vi "DataPathDialog.vi"(11 "Path":path=path "click on the folder icon to choose a folder") -> (1 "canceled?":bool, 3 "Path out":path)   [LabVIEW 2022 SP3]
panel:
  in  "Cancel Button":bool
  in  "OK Button":bool
  # "Welcome to Oberlin Acoustics \nacquiring data from a violin"
  # "1. Select your Data Folder\n       this is the folder for all your data"
  # "2. Check out directions\n       understand where to get help"
  # "https://sites.google.com/view/oberlinacoustics"
  # "3. Getting Started\n       First time users should hit the Getting     \n       Started button on the next screen (after \n       clicking on OK)"
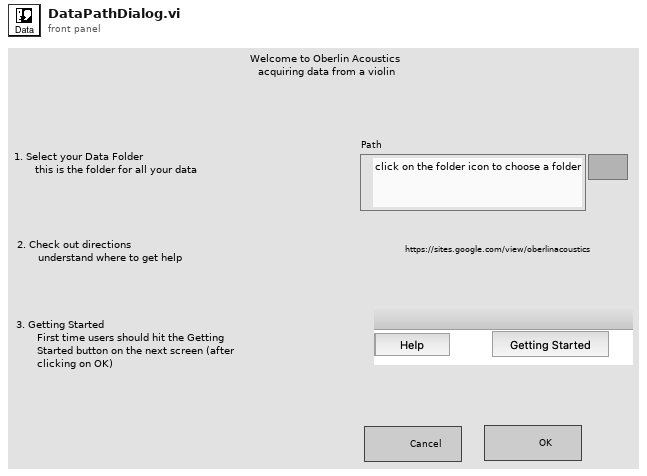
[diagram p1: front panel]
types:
  T1 = enum8{"Enabled", "Disabled", "Disabled and Grayed Out"}
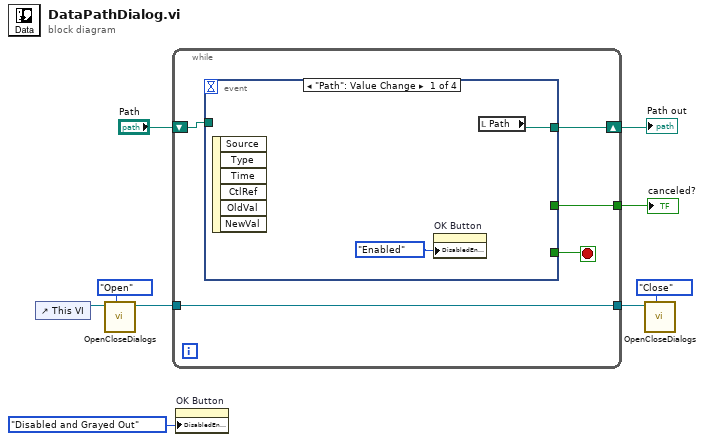
[diagram p0: block diagram]
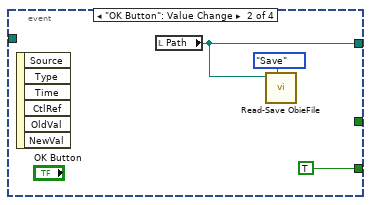
[diagram p2: hidden frame]
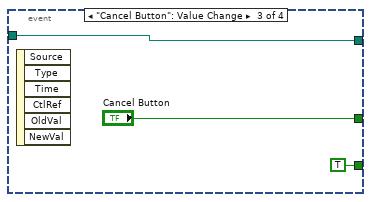
[diagram p3: hidden frame]
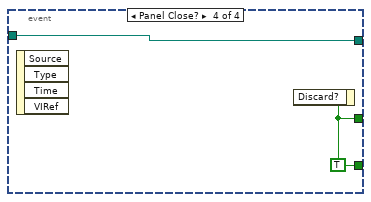
[diagram p4: hidden frame]
diagram:
  n1 = control-ref of="This VI"() -> (w4:refnum<vi>)
  n2 = call "OpenCloseDialogs.vi"("Task"=enum16{"Open", "Close"}."Open", "VI in"=w4) -> ("VI out"=w1:refnum<vi>)  [unwired: 8 in, 1 out]
  n3 = while {
    shift-right: [w12] -> w9
    shift-left: "Path" -> [w14]
    tunnel: [w11] -> w7
    tunnel: [w10] -> w2
    tunnel: w1 -> [w10]
    stop <- w13 stop-if-true
    n4 = event shown="[0] \"Path\": Value Change" {
      selector: _ -> [_ _ _ _]
      dyn-events: _ -> [_ _ _ _]
      timeout: _ -> [_ _ _ _]
      tunnel: [w16 w19 w22 w24] -> w12
      tunnel: w14 -> [_ _ w22 w24]
      tunnel: [_ TRUE TRUE w23] -> w13
      tunnel: [_ _ "Cancel Button" w23] -> w11
      event "Path": Value Change {
        n5 = event-data() -> ()  [unwired: 1 in, 6 out]
        n6 = property on="OK Button" class="Bool"("DisabledEnum"=T1."Enabled" ("Disabled")) -> ()  [unwired: 2 in, 2 out]
        n7 = local read "Path"() -> (w16:path)
      }
      event "OK Button": Value Change {
        n8 = event-data() -> ()  [unwired: 1 in, 6 out]
        n9 = local read "Path"() -> (w19:path)
        n10 = call "Read-Save ObieFile.vi"("Task"=enum16{"Save", "Read"}."Save", "DataPath"=w19) -> ()  [unwired: 7 in, 3 out]
      }
      event "Cancel Button": Value Change {
        n11 = event-data() -> ()  [unwired: 1 in, 6 out]
      }
      event Panel Close? {
        w23 = TRUE
        n12 = event-data() -> ()  [unwired: 1 in, 4 out]
        n13 = event-data("Discard?"=w23) -> ()  [unwired: 1 in, 1 out]
      }
    }
  }
  "Path out" <- w9
  "canceled?" <- w7
  n14 = property on="OK Button" class="Bool"("DisabledEnum"=T1."Disabled and Grayed Out" ("Disabled")) -> ()  [unwired: 2 in, 2 out]
  n15 = call "OpenCloseDialogs.vi"("Task"=enum16{"Open", "Close"}."Close", "VI in"=w2) -> ()  [unwired: 8 in, 2 out]
